vi "Request Frame.vi"(7 "Ignore Response":bool, 8 "error in (no error)":errorcluster, 9 "DA":u8, 10 "PGN":u32, 11 "connection info":T1) -> (0 "error out":errorcluster, 2 "Response Frame":T3 {"payload" format="%x"; "timestamp" format="%<%.7X\n%x>T"; "type" items=["CAN Data"=0, "CAN Remote"=1, "CAN Bus Error"=2, "CAN 2.0 Data"=8, "CAN FD Data"=16, "CAN FD+BRS Data"=24, "J1939 Data"=192, "Delay"=224, "Log Trigger"=225, "Start Trigger"=226]; "identifier" format="%x"}, 3 "connection info":T1)   [LabVIEW 2019, in "J1939 Workspace Shared.lvlib"]
uses:
  J1939 Workspace Shared.lvlib
  <vilib>/xnet/xnet.llb/XNET Frame CAN.ctl
  <vilib>/xnet/xnet.llb/XNET Frame Type CAN.ctl
  <vilib>/NI/STM/TCP/TCP Connection Info.ctl
  <vilib>/NI/STM/SubVIs/MetaDataElement.ctl
  Addon/Addon Shared/Types/Request Message.ctl
  Addon/Addon Shared/J1939 Addon Shared.lvlib
  <vilib>/NI/NI VeriStand Addon Network Comm/Shared/NI VeriStand Addon Network Comm Shared.lvlib
  <vilib>/NI/STM/NI STM.lvlib
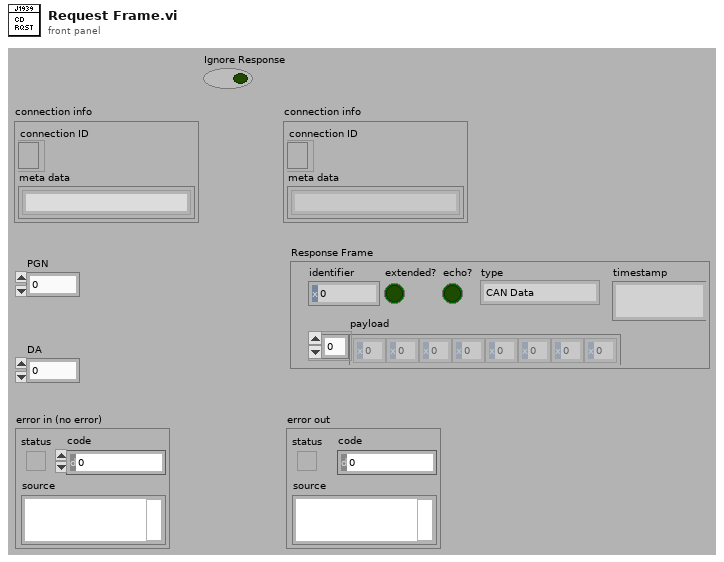
[diagram p1: front panel]
types:
  T1 = typedef "NI STM.lvlib/TCP Connection Info.ctl" = cluster{"connection ID":refnum<k5>, "meta data":T2[]}
  T2 = typedef "NI STM.lvlib/MetaDataElement.ctl" = string
  T3 = typedef "XNET Frame CAN.ctl" = cluster{"timestamp":timestamp, "payload":u8[], "identifier":u32, "type":T4, "extended?":bool, "echo?":bool}
  T4 = typedef "XNET Frame Type CAN.ctl" = u8
  T5 = typedef "J1939 Addon Shared.lvlib/Request Message.ctl" = cluster{"PGN":u32, "DA":u8, "Ignore Response":bool}
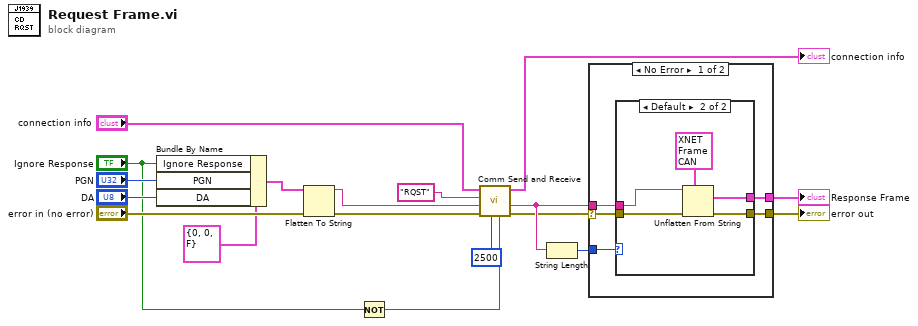
[diagram p0: block diagram]
diagram:
  n1 = Bundle By Name(cluster=T5 {"PGN"=0, "DA"=0, "Ignore Response"=FALSE} ("Cluster"), "Ignore Response"="Ignore Response", "PGN"="PGN", "DA"="DA") -> (w11:T5)
  n2 = Flatten To String(anything=w11, error in (no error)="error in (no error)") -> (data string=w8:string, error out=w7:errorcluster)  [unwired: 2 in, 1 out]
  n3 = Not(x="Ignore Response") -> (.not. x?=w1:bool)
  n4 = call <vilib>:"Comm Send and Receive.vi"("Resp Required?"=w1, "Timeout (ms)"=u32 2500 ("Timeout ms (5000)"), "error in (no error)"=w7, "Data"=w8, "Name"="RQST" ("Command"), "connection info"="connection info") -> ("error out"=w3:errorcluster, "Data"=w5:string, "connection info"=→"connection info":T1)  [unwired: 2 in, 1 out]
  n5 = String Length(string=w5) -> (length=w18:i32)
  n6 = case shown="No Error" w3 {
    selector: w3 -> [w20 w30]
    tunnel: [w23 w30] -> w15
    tunnel: w18 -> [w22 _]
    tunnel: w5 -> [w21 _]
    tunnel: [w19 _] -> w17
    frame No Error {
      n7 = case shown="Default" w22 {
        tunnel: w20 -> [w24 w28]
        tunnel: w21 -> [_ w25]
        tunnel: [w24 w27] -> w23
        tunnel: [_ w26] -> w19
        frame 0 {
        }
        frame Default {
          n8 = Unflatten From String(type=T3 {"timestamp"=timestamp(0 s since 1904-01-01), "payload"=[], "identifier"=0, "type"=0, "extended?"=FALSE, "echo?"=FALSE} ("element"), binary string=w25, error in (no error)=w28) -> (value=w26:T3, error out=w27:errorcluster)  [unwired: 2 in, 1 out]
        }
      }
    }
    frame Error {
    }
  }
  "Response Frame" <- w17
  "error out" <- w15
